vi "numbers.vi"() -> ()   [LabVIEW 2021, in "Ceyear.lvlib"]
uses:
  <instrlib>/Ceyear/Ceyear.lvlib
panel:
  out "VISA resource name out":refnum<visa-resource-name>
  out "error out":errorcluster
  in  "error in (no error)":errorcluster
  in  "VISA resource name":refnum<visa-resource-name>
  out "Array Data":dbl[](array[numeric]) format="%.2f"
  in  "String":string
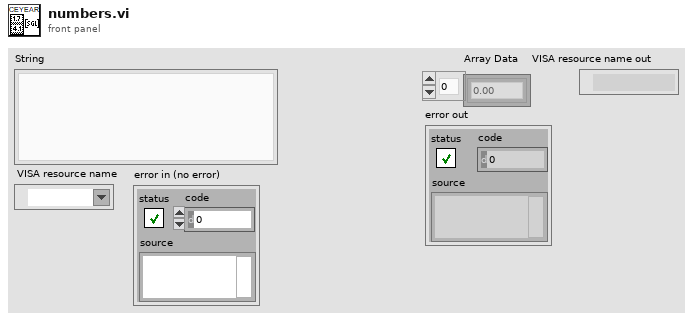
[diagram p1: front panel]
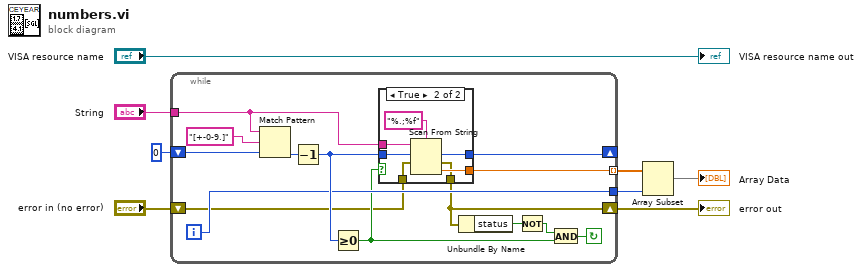
[diagram p0: block diagram]
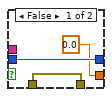
[diagram p2: hidden frame]
diagram:
  n1 = while {
    tunnel: "String" -> [w17]
    tunnel: [w18] -> w4
    tunnel: [w15] -> w7 mode=indexing
    shift-left: 0 -> [w21]
    shift-right: [w16] -> _
    shift-right: [w10] -> w1
    shift-left: "error in (no error)" -> [w12]
    i -> [w18]
    stop <- w14 continue-if-true
    n2 = Match Pattern(string=w17, regular expression="[+-0-9.]", offset (0)=w21) -> (offset past match=w20:i32)  [unwired: 3 out]
    n3 = Decrement(x=w20) -> (x-1=w19:i32)
    n4 = Greater Or Equal To 0?(x=w19) -> (x >= 0?=w13:bool)
    n5 = case shown="True" w13 {
      tunnel: w19 -> [w25 w32]
      tunnel: w17 -> [_ w31]
      tunnel: [w25 w30] -> w16
      tunnel: [0.0 w29] -> w15
      tunnel: w12 -> [w24 w28]
      tunnel: [w24 w27] -> w10
      frame False {
      }
      frame True {
        n6 = Scan From String(format string="%.;%f", input string=w31, initial scan location=w32, error in=w28) -> (offset past scan=w30:u32, error out=w27:errorcluster, output 1=w29:dbl)  [unwired: 1 in, 1 out]
      }
    }
    n7 = Unbundle By Name(w10) -> ("status"=w11:bool)
    n8 = Not(x=w11) -> (.not. x?=w9:bool)
    n9 = And(x=w9, y=w13) -> (x .and. y?=w14:bool)
  }
  "error out" <- w1
  n10 = Array Subset(array=w7, length=w4) -> (→"Array Data":dbl[])  [unwired: 1 in]
  "VISA resource name out" <- "VISA resource name"
